vi "mod_Loop Filter.vi"(0 "x(n)":dbl, 5 "reverse coefficients":dbl[](array[numeric]), 7 "forward coefficients":dbl[](array[numeric]), 11 "error in (no error)":errorcluster, 13 "reset ? (T)":bool=TRUE) -> (4 "y(n)":dbl, 15 "error out":errorcluster)   [LabVIEW 2020, in "niAMT.lvlib"]
uses:
  <vilib>/addons/Modulation/niAMT.lvlib
  <vilib>/ptbypt/NI_PtbyPt.lvlib
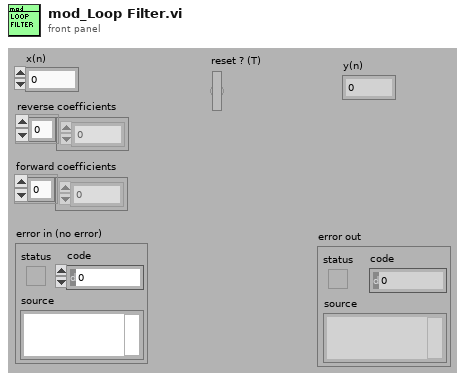
[diagram p1: front panel]
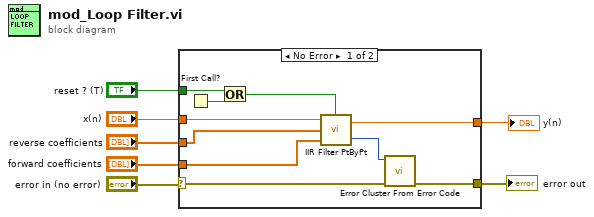
[diagram p0: block diagram]
diagram:
  n1 = case shown="No Error" "error in (no error)" {
    selector: "error in (no error)" -> [w10 w18]
    tunnel: "reset ? (T)" -> [w17 _]
    tunnel: "x(n)" -> [w15 _]
    tunnel: "reverse coefficients" -> [w14 _]
    tunnel: "forward coefficients" -> [w13 _]
    tunnel: [w11 _] -> w3
    tunnel: [w8 w18] -> w1
    frame No Error {
      n2 = First Call?() -> (First Call?: T/F=w16:bool)
      n3 = Or(x=w17, y=w16) -> (x .or. y?=w12:bool)
      n4 = call <vilib>:"IIR Filter PtByPt.vi"("initialize"=w12, "Forward Coefficients"=w13, "Reverse Coefficients"=w14, "x"=w15) -> ("error"=w9:i32, "Filtered x"=w11:dbl)
      n5 = call <vilib>:"Error Cluster From Error Code.vi"("error in (no error)"=w10, "error code (0)"=w9) -> ("error out"=w8:errorcluster)  [unwired: 1 in, 6 out]
    }
    frame Error {
    }
  }
  "y(n)" <- w3
  "error out" <- w1
